vi "Close and Save Opened VIS.vi"(8 "error in":errorcluster, 10 "Save?":bool, 11 "Project in":refnum<class "Project.lvclass">) -> (0 "error out":errorcluster)   [LabVIEW 2020, in "Panther Dashboard.lvlib"]
uses:
  Panther Dashboard.lvlib
  Class/Project/Project.lvclass
  Class/Project/Project.lvclass/Project.ctl
  Class/Project/Read Target Ref.vi
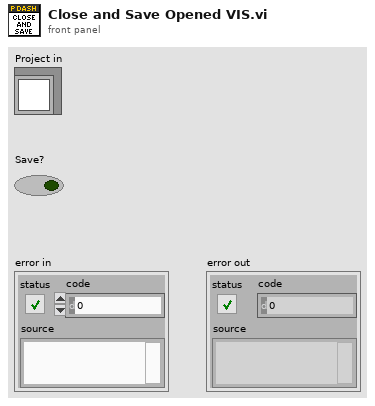
[diagram p1: front panel]
types:
  T1 = enum32{"Invalid", "Standard", "Closed", "Hidden", "Minimized", "Maximized"}
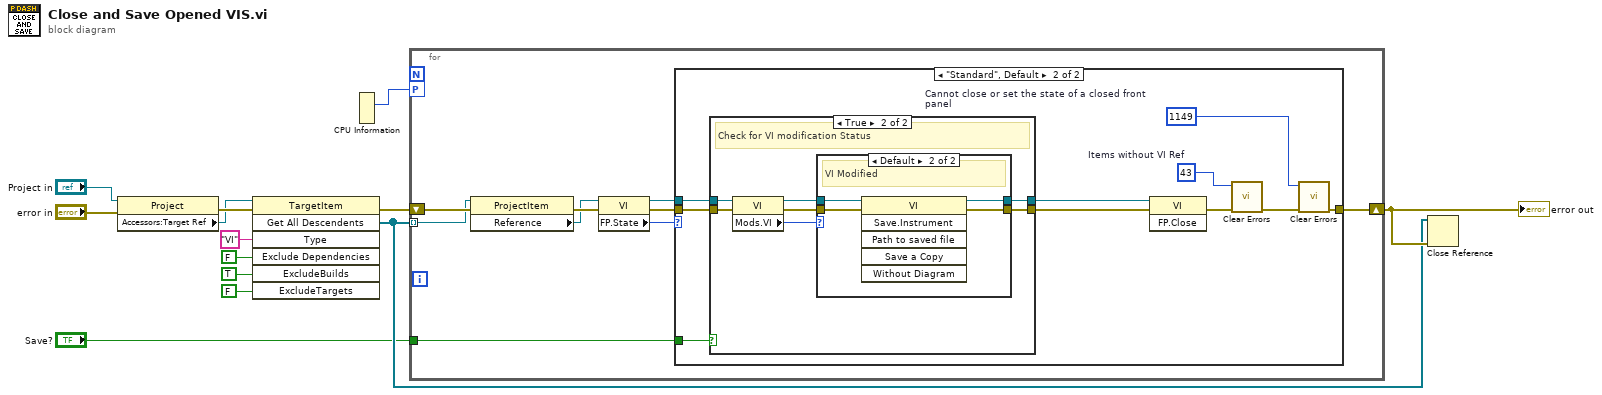
[diagram p0: block diagram]
diagram:
  n1 = property class="Project"(reference="Project in", error in="error in") -> (error out=w11:errorcluster, "Accessors:Target Ref"=w3:refnum<vi>)  [unwired: 1 out]
  n2 = invoke class="TargetItem" method="Get All Descendents"(reference=w3, error in=w11, "Type"="VI", "Exclude Dependencies"=FALSE ("ExcludeDependencies"), "ExcludeBuilds"=TRUE, "ExcludeTargets"=FALSE) -> (error out=w10:errorcluster, "All Descendents"=w4:refnum<vi>[])  [unwired: 1 in, 5 out]
  n3 = CPU Information() -> (5:w1:i32)  [unwired: 3 out]
  n4 = for {
    tunnel: w4 -> [w19] mode=indexing
    shift-right: [w20] -> w12
    shift-left: w10 -> [w22]
    tunnel: "Save?" -> [w18]
    workers-P: w1 -> [_]
    n5 = property class="ProjectItem"(reference=w19, error in=w22) -> (error out=w21:errorcluster, "Reference"=w16:refnum<vi>)  [unwired: 1 out]
    n6 = property class="VI"(reference=w16, error in=w21) -> (reference out=w15:refnum<vi>, error out=w17:errorcluster, "FP.State"=w14:T1)
    n7 = case shown="\"Standard\", Default" w14 {
      tunnel: [w23 w31] -> w20
      tunnel: w18 -> [_ w26]
      tunnel: w17 -> [w23 w25]
      tunnel: w15 -> [_ w24]
      frame "Closed" {
      }
      frame "Standard", Default {
        w28 = 1149  # Cannot close or set the state of a closed front panel
        w29 = 43  # Items without VI Ref
        n8 = case shown="True" w26 {
          tunnel: w25 -> [w35 w42]
          tunnel: w24 -> [w34 w39]
          tunnel: [w34 w36] -> w27
          tunnel: [w35 w40] -> w30
          frame False {
            # "No Save"
          }
          frame True {
            # "Check for VI modification Status"
            n9 = property class="VI"(reference=w39, error in=w42) -> (reference out=w37:refnum<vi>, error out=w41:errorcluster, "Mods.VI"=w38:u64)
            n10 = case shown="Default" w38 {
              tunnel: w41 -> [w44 w48]
              tunnel: w37 -> [w43 w46]
              tunnel: [w43 w45] -> w36
              tunnel: [w44 w47] -> w40
              frame 0 {
                # "No changes"
              }
              frame Default {
                # "VI Modified"
                n11 = invoke class="VI" method="Save.Instrument"(reference=w46, error in=w48) -> (reference out=w45:refnum<vi>, error out=w47:errorcluster)  [unwired: 4 in, 4 out]
              }
            }
          }
        }
        n12 = invoke class="VI" method="FP.Close"(reference=w27, error in=w30) -> (error out=w33:errorcluster)  [unwired: 1 in, 2 out]
        n13 = call <vilib>:"Clear Errors.vi"("error in (no error)"=w33, "specific error code to clear (0: all)"=w29) -> ("error out"=w32:errorcluster)  [unwired: 4 in, 1 out]
        n14 = call <vilib>:"Clear Errors.vi"("error in (no error)"=w32, "specific error code to clear (0: all)"=w28) -> ("error out"=w31:errorcluster)  [unwired: 4 in, 1 out]
      }
    }
  }
  "error out" <- w12
  n15 = Close Reference(reference=w4, error in (no error)=w12) -> ()  [unwired: 1 out]
